vi "SyncLoop.vi"(8 "error in (no error)":errorcluster, 11 "PXI_MultiTrig in":refnum<class "PXI_MultiTrig.lvclass">) -> (0 "error out":errorcluster, 1 "Locked":bool, 2 "Time Ref Offset (ns)":dbl format="%#_12f", 3 "PXI_MultiTrig out":refnum<class "PXI_MultiTrig.lvclass">, 4 "LostLock":bool, 6 "ObtainLock":bool)   [LabVIEW 2018, in "SyncPlugins.lvlib" / "PXI_MultiTrig.lvclass"]
uses:
  PXI_MultiTrig.lvclass
  X:/Projects/PMUCal/Modules/Sync/SyncPlugins/SyncPluginBase/SyncPluginBase.lvclass
  SyncPluginBase/SyncPluginBase.lvclass/SyncPluginBase.ctl
  PXI_MultiTrig.lvclass/PXI_MultiTrig.ctl
  Typedefs/clClocks.ctl
  SyncPluginBase/Accessors/Write Locked.vi
  SyncPluginBase/Accessors/Write LostLock.vi
  Accessors/Read SyncWindowsClock.vi
  Accessors/Read RefClkSession.vi
  SyncPluginBase/Accessors/Write PPSTime.vi
  SyncPluginBase/Accessors/Read Run.vi
  Accessors/Read TimingSession.vi
  SyncPluginBase/Accessors/Read Initiated.vi
  SyncPluginBase/Accessors/Read Locked.vi
  SyncPluginBase/Accessors/Read Clocks.vi
  <instrlib>/niSync/niSync.llb/niSync Read Trigger Time Stamp (Single).vi
  SyncPluginBase/SyncPluginBase.lvclass
panel:
  out "RefClk Present":bool
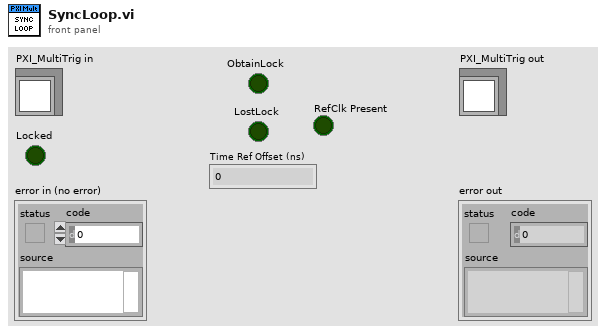
[diagram p1: front panel]
types:
  T1 = typedef "SyncPlugins.lvlib/PXI_MultiTrig.lvclass/clClocks.ctl" = cluster{"Name":string, "RefClk":string, "ClkTerminal":string, "Frequency":dbl, "DutyCycle":dbl, "ClkType":string, "Initiated":bool, "TrigTime":bool, "Delay":dbl}
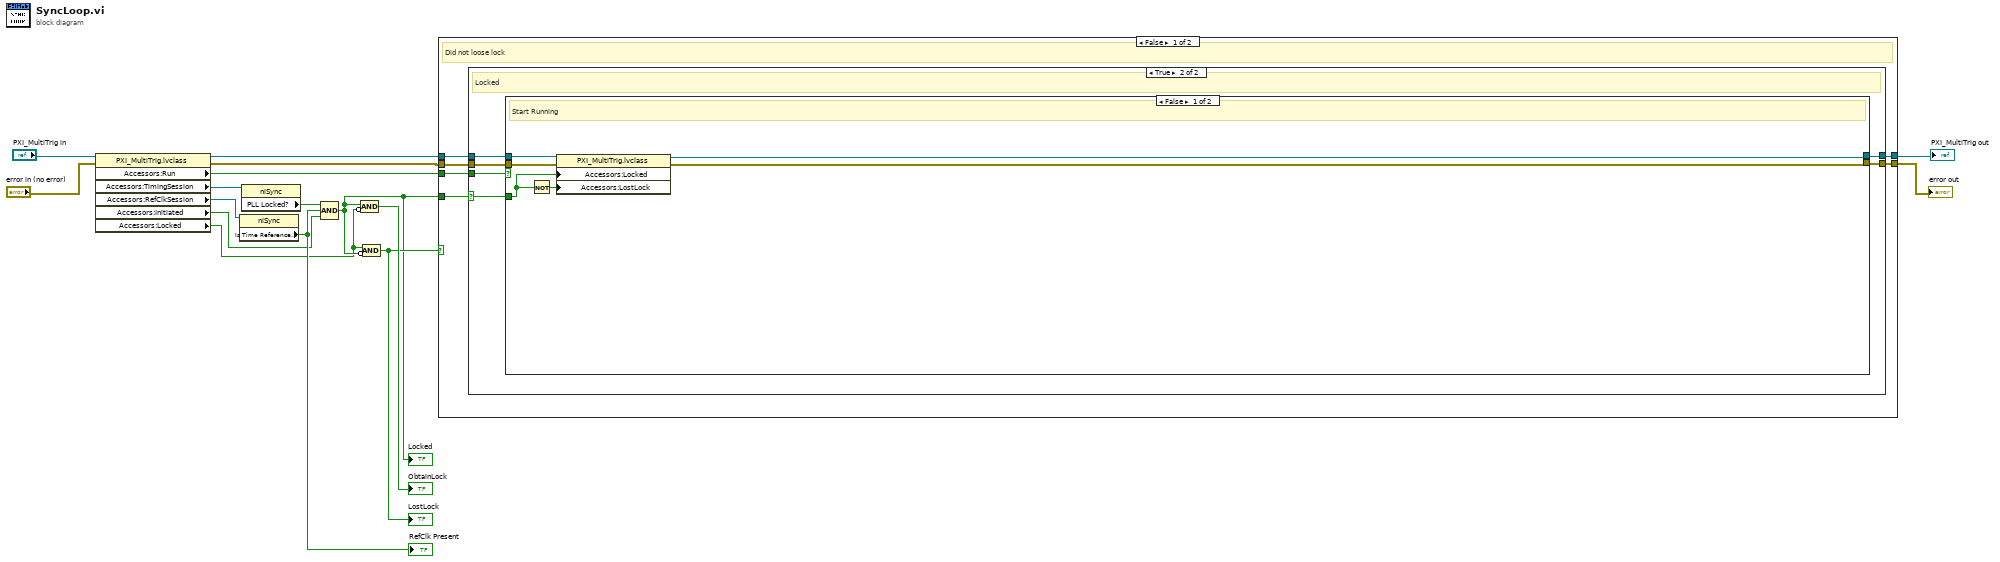
[diagram p0: block diagram]
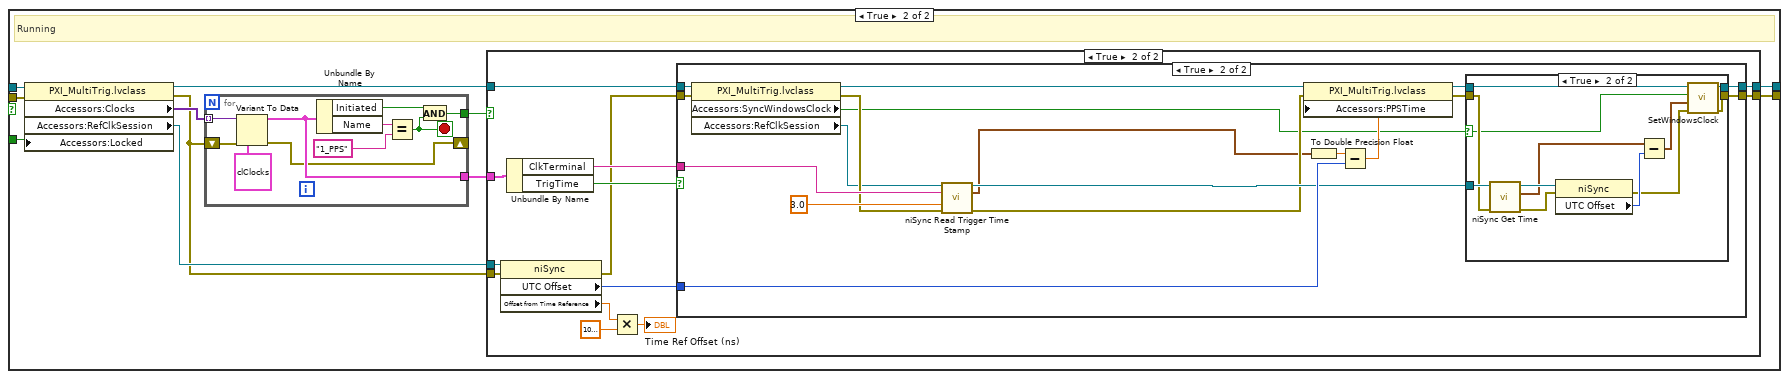
[diagram p3: hidden frame]
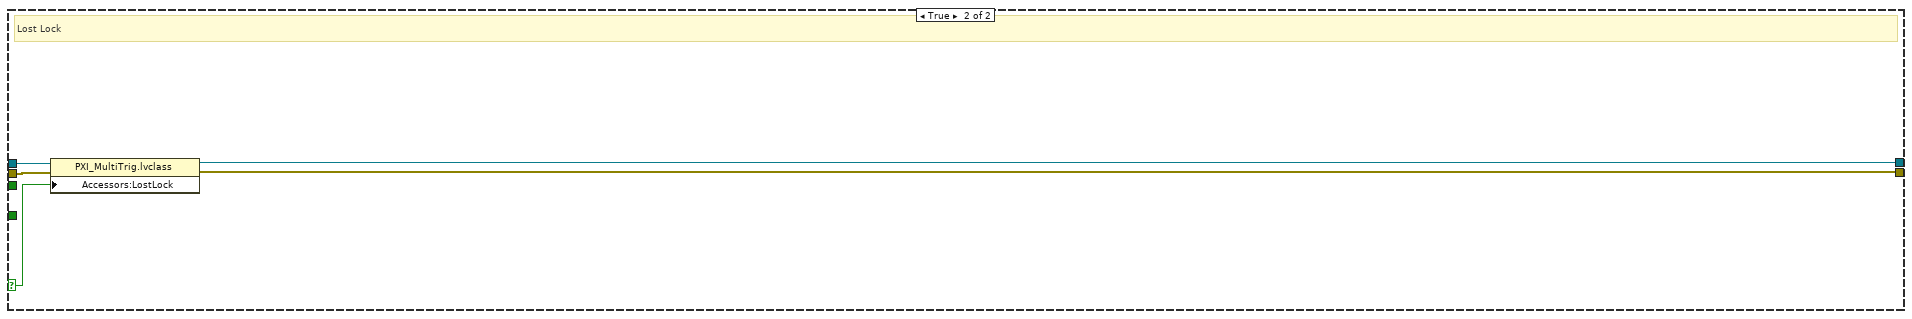
[diagram p7: hidden frame]
diagram:
  n1 = property class="PXI_MultiTrig.lvclass"(reference="PXI_MultiTrig in", error in="error in (no error)") -> (reference out=w10:refnum<class "PXI_MultiTrig.lvclass">, error out=w8:errorcluster, "Accessors:Run"=w7:bool, "Accessors:TimingSession"=w12:refnum<k15>, "Accessors:RefClkSession"=w3:refnum<k15>, "Accessors:Initiated"=w1:bool, "Accessors:Locked"=w2:bool)
  n2 = property class="niSync"(reference=w3) -> ("Is Time Reference Present"=w4:bool)  [unwired: 1 in, 2 out]
  "RefClk Present" <- w4
  n3 = property class="niSync"(reference=w12) -> ("PLL Locked?"=w6:bool)  [unwired: 1 in, 2 out]
  n4 = Compound Arithmetic op=AND(w6, w4, w1) -> (w5:bool)
  "Locked" <- w5
  n5 = Compound Arithmetic op=AND(w5, invert w2) -> (→"ObtainLock":bool)
  n6 = Compound Arithmetic op=AND(w2, invert w5) -> (w9:bool)
  "LostLock" <- w9
  n7 = case shown="False" w9 {
    selector: w9 -> [_ w109]
    tunnel: [w22 w108] -> w16
    tunnel: [w17 w107] -> w15
    tunnel: w10 -> [w20 w111]
    tunnel: w8 -> [w19 w110]
    tunnel: w5 -> [w21 _]
    tunnel: w7 -> [w18 _]
    frame False {
      # "Did not loose lock"
      n8 = case shown="True" w21 {
        selector: w21 -> [_ w25]
        tunnel: [w24 w30] -> w22
        tunnel: w20 -> [w24 w29]
        tunnel: w19 -> [w23 w28]
        tunnel: w18 -> [_ w27]
        tunnel: [w23 w26] -> w17
        frame False {
          # "Not yet locked"
        }
        frame True {
          # "Locked"
          n9 = case shown="False" w27 {
            tunnel: [w34 w43] -> w30
            tunnel: w29 -> [w36 w47]
            tunnel: w28 -> [w35 w46]
            tunnel: [w33 w40] -> w26
            tunnel: w25 -> [w32 w39]
            frame False {
              # "Start Running"
              n10 = Not(x=w32) -> (.not. x?=w31:bool)
              n11 = property class="PXI_MultiTrig.lvclass"(reference=w36, error in=w35, "Accessors:Locked"=w32, "Accessors:LostLock"=w31) -> (reference out=w34:refnum<class "PXI_MultiTrig.lvclass">, error out=w33:errorcluster)
            }
            frame True {
              # "Running"
              n12 = property class="PXI_MultiTrig.lvclass"(reference=w47, error in=w46, "Accessors:Locked"=w39) -> (reference out=w44:refnum<class "PXI_MultiTrig.lvclass">, error out=w37:errorcluster, "Accessors:Clocks"=w45:variant[], "Accessors:RefClkSession"=w38:refnum<k15>)
              n13 = for {
                tunnel: w45 -> [w101] mode=indexing
                tunnel: [w98] -> w42
                tunnel: [w102] -> w41
                shift-right: [w97] -> _
                shift-left: w37 -> [w100]
                stop <- w104 stop-if-true
                n14 = Variant To Data(error in=w100, type=T1 {"Name"="", "RefClk"="/PXI1Slot7/PFI1", "ClkTerminal"="PXI_Star4", "Frequency"=0.0, "DutyCycle"=0.0, "ClkType"="", "Initiated"=FALSE, "TrigTime"=FALSE, "Delay"=0.0} ("clClocks"), Variant=w101) -> (data=w98:T1, error out=w97:errorcluster)
                n15 = Unbundle By Name(w98) -> ("Initiated"=w103:bool, "Name"=w106:string)
                n16 = Equal?(x=w106, y="1_PPS") -> (x = y?=w104:bool)
                n17 = And(x=w103, y=w104) -> (x .and. y?=w102:bool)
              }
              n18 = case shown="True" w41 {
                tunnel: w44 -> [w49 w62]
                tunnel: [w49 w61] -> w43
                tunnel: w42 -> [_ w60]
                tunnel: [w48 w58] -> w40
                tunnel: w37 -> [w48 w56]
                tunnel: w38 -> [_ w54]
                frame False {
                }
                frame True {
                  n19 = property class="niSync"(reference=w54, error in=w56) -> (error out=w55:errorcluster, "UTC Offset"=w53:i32, "Offset from Time Reference"=w52:dbl)  [unwired: 1 out]
                  n20 = Unbundle By Name(w60) -> ("ClkTerminal"=w59:string, "TrigTime"=w57:bool)
                  n21 = Multiply(x=w52, y=1000000000.0) -> (x*y=→"Time Ref Offset (ns)":dbl)
                  n22 = case shown="True" w57 {
                    tunnel: w62 -> [w64 w82]
                    tunnel: [w64 w71] -> w61
                    tunnel: w59 -> [_ w81]
                    tunnel: w53 -> [_ w78]
                    tunnel: w55 -> [w63 w76]
                    tunnel: [w63 w70] -> w58
                    frame False {
                    }
                    frame True {
                      n23 = property class="PXI_MultiTrig.lvclass"(reference=w82, error in=w76) -> (reference out=w72:refnum<class "PXI_MultiTrig.lvclass">, error out=w75:errorcluster, "Accessors:SyncWindowsClock"=w66:bool, "Accessors:RefClkSession"=w73:refnum<k15>)
                      n24 = call-poly <instrlib>:"niSync Read Trigger Time Stamp.vi"("instrument handle"=w73, "terminal"=w81, "timeout"=3.0, "error in (no error)"=w75) -> ("instrument handle out"=w74:refnum<k15>, "time stamp out"=w65:timestamp, "error out"=w69:errorcluster)  [unwired: 8 in, 1 out]
                      n25 = To Double Precision Float(number=w65) -> (double precision float=w79:dbl)
                      n26 = Subtract(x=w79, y=w78) -> (x-y=w77:dbl)
                      n27 = property class="PXI_MultiTrig.lvclass"(reference=w72, error in=w69, "Accessors:PPSTime"=w77) -> (reference out=w67:refnum<class "PXI_MultiTrig.lvclass">, error out=w68:errorcluster)
                      n28 = case shown="True" w66 {
                        selector: w66 -> [_ w85]
                        tunnel: w74 -> [_ w96]
                        tunnel: [w84 w90] -> w71
                        tunnel: [w83 w89] -> w70
                        tunnel: w68 -> [w83 w88]
                        tunnel: w67 -> [w84 w87]
                        frame False {
                        }
                        frame True {
                          n29 = call <instrlib>:"niSync Get Time.vi"("error in (no error)"=w88, "instrument handle"=w96) -> ("error out"=w92:errorcluster, "time"=w93:timestamp, "instrument handle out"=w95:refnum<k15>)  [unwired: 5 in]
                          n30 = property class="niSync"(reference=w95, error in=w92) -> (error out=w86:errorcluster, "UTC Offset"=w94:i32)  [unwired: 1 out]
                          n31 = Subtract(x=w93, y=w94) -> (x-y=w91:timestamp)
                          n32 = call "SetWindowsClock.vi"("error in (no error)"=w86, "time stamp"=w91, "SyncWinClk"=w85, "SyncPluginBase in"=w87) -> ("error out"=w89:errorcluster, "SyncPluginBase out"=w90:refnum<class "PXI_MultiTrig.lvclass">)  [unwired: 6 in]
                        }
                      }
                    }
                  }
                }
              }
            }
          }
        }
      }
    }
    frame True {
      # "Lost Lock"
      n33 = property class="PXI_MultiTrig.lvclass"(reference=w111, error in=w110, "Accessors:LostLock"=w109) -> (reference out=w108:refnum<class "PXI_MultiTrig.lvclass">, error out=w107:errorcluster)
    }
  }
  "error out" <- w15
  "PXI_MultiTrig out" <- w16
